vi "Initialization.vi"() -> (0 "Devices":string[](array[string]), 2 "Video formats":string[](array[string]), 3 "Initialization Out":refnum<k7>)   [LabVIEW 2009]
panel:
  in  "ICImagingControl":refnum<k7>(container)
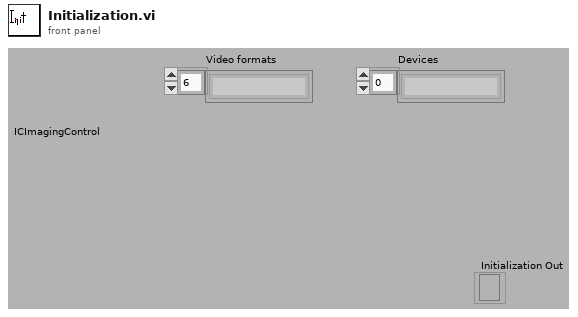
[diagram p1: front panel]
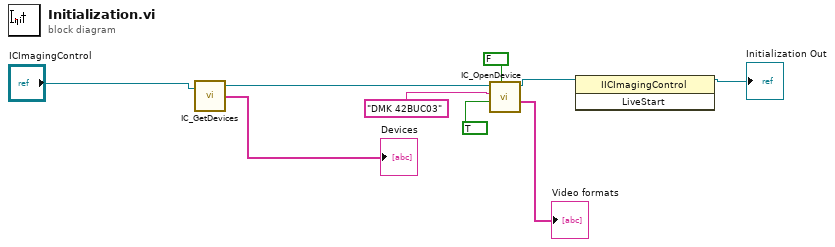
[diagram p0: block diagram]
diagram:
  n1 = call <userlib>:"IC_GetDevices.vi"("ICImagingControl In"="ICImagingControl") -> ("ICImagingControl Out"=w7:refnum<k7>, "Devices"=→"Devices":string[])  [unwired: 1 in, 1 out]
  n2 = call <userlib>:"IC_OpenDevice.vi"("Color"=FALSE, "Live"=TRUE, "Device"="DMK 42BUC03", "ICImagingControl In"=w7) -> ("VideoFormats"=→"Video formats":string[], "ICImagingControl Out"=w2:refnum<k7>)  [unwired: 2 in, 4 out]
  n3 = invoke class="IICImagingControl" method="LiveStart"(reference=w2) -> (reference out=→"Initialization Out":refnum<k7>)  [unwired: 2 in, 2 out]
